vi "ex_GetOneLineFromChunk.vi"(8 "error in (no error)":errorcluster, 9 "file_params":T1 {"time preference" items=["Absolute", "Relative"]; "x_columns" items=["None", "One", "Multiple"]}, 10 "current chunk":string, 11 "file refs in":T2={"file ref"=refnum, "file size (bytes:0)"=0, "read pointer (bytes:0)"=0, "chunk size (bytes:65000)"=65000}) -> (0 "error out":errorcluster, 1 "line":string, 2 "chunk out":string, 3 "dup file refs":T2={"file ref"=refnum, "file size (bytes:0)"=0, "read pointer (bytes:0)"=0, "chunk size (bytes:65000)"=65000}, 4 "end-of-file?":bool)   [LabVIEW 2017]
uses:
  <vilib>/express/express shared/ExFile.llb/ex_FileReference.ctl
  <vilib>/express/express input/ExFileReadBlock.llb/ex_ReadFileParams.ctl
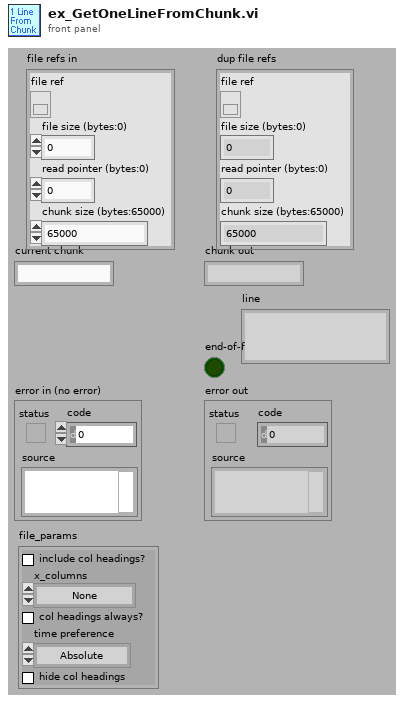
[diagram p1: front panel]
types:
  T1 = typedef "ex_ReadFileParams.ctl" = cluster{"include col headings?":bool, "x_columns":u16, "col headings always?":bool, "time preference":u16, "hide col headings":bool}
  T2 = typedef "ex_FileReference.ctl" = cluster{"file ref":refnum<file>, "file size (bytes:0)":i32, "read pointer (bytes:0)":i32, "chunk size (bytes:65000)":i32}
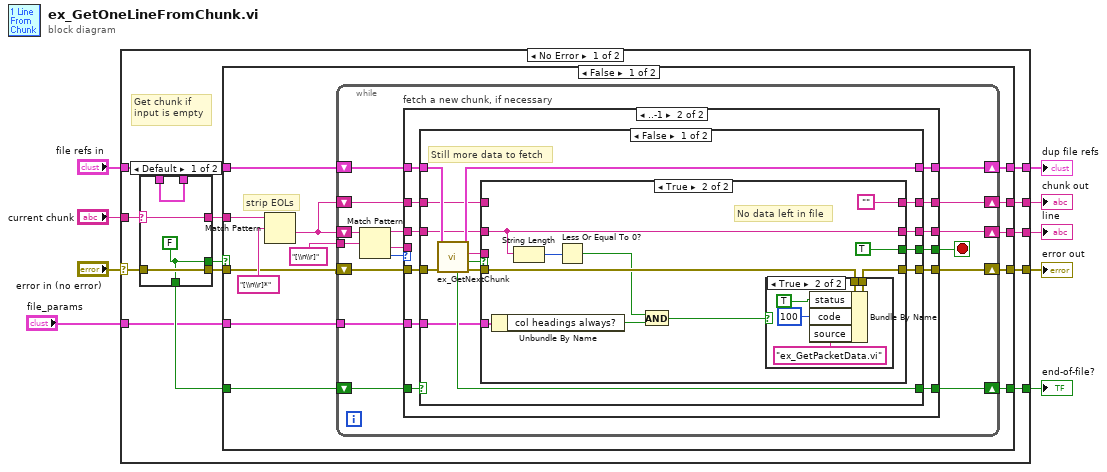
[diagram p0: block diagram]
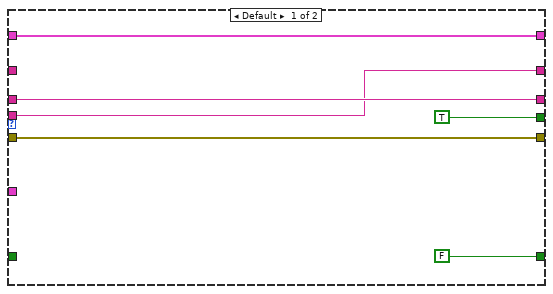
[diagram p2: hidden frame]
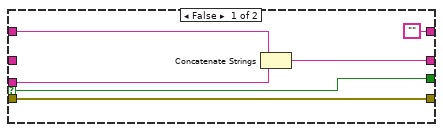
[diagram p3: hidden frame]
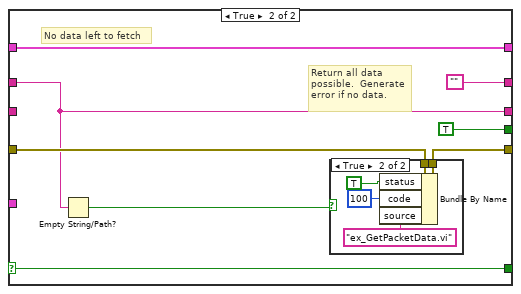
[diagram p5: hidden frame]
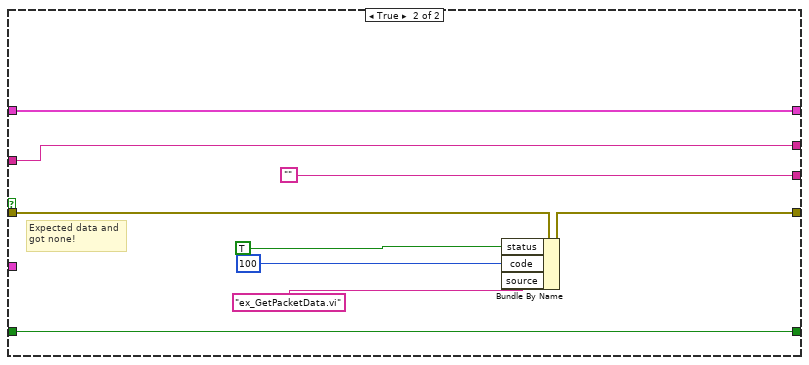
[diagram p7: hidden frame]
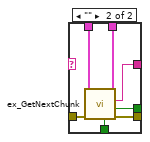
[diagram p8: hidden frame]
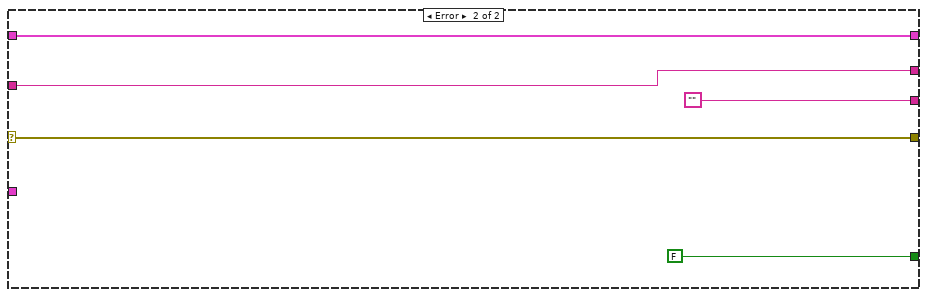
[diagram p9: hidden frame]
diagram:
  n1 = case shown="No Error" "error in (no error)" {
    selector: "error in (no error)" -> [w16 w144]
    tunnel: "current chunk" -> [w18 w145]
    tunnel: [w23 w145] -> w7
    tunnel: [w19 w144] -> w6
    tunnel: [w22 ""] -> w5
    tunnel: [w21 w143] -> w4
    tunnel: "file refs in" -> [w14 w143]
    tunnel: [w20 FALSE] -> w2
    tunnel: "file_params" -> [w10 _]
    frame No Error {
      # "Get chunk if\ninput is empty"
      n2 = case shown="Default" w18 {
        selector: w18 -> [w132 _]
        tunnel: [w132 w136] -> w17
        tunnel: w16 -> [w131 w140]
        tunnel: w14 -> [w133 w139]
        tunnel: [w133 w138] -> w15
        tunnel: [w131 w137] -> w13
        tunnel: [w130 w135] -> w12
        tunnel: [w130 w134] -> w11
        frame Default {
          w130 = FALSE ("no data error")
        }
        frame "" {
          n3 = call <vilib>:"ex_GetNextChunk.vi"("error in (no error)"=w140, "file refs"=w139) -> ("error out"=w137:errorcluster, "no data error"=w135:bool, "chunk"=w136:string, "dup file refs"=w138:T2, "end-of-file?"=w134:bool)  [unwired: 3 in, 2 out]
        }
      }
      n4 = case shown="False" w12 {
        tunnel: [w34 w122] -> w23
        tunnel: [w33 ""] -> w22
        tunnel: [w32 w123] -> w21
        tunnel: [w26 w124] -> w20
        tunnel: [w31 w125] -> w19
        tunnel: w17 -> [w29 w122]
        tunnel: w15 -> [w28 w123]
        tunnel: w13 -> [w27 w126]
        tunnel: w11 -> [w25 w124]
        tunnel: w10 -> [w24 _]
        frame False {
          # "strip EOLs"
          n5 = Match Pattern(string=w29, regular expression="[\\n\\r]*") -> (after substring=w36:string)  [unwired: 4 out]
          n6 = while {
            shift-right: [w44] -> w34
            shift-left: w36 -> [w47]
            shift-right: [w45] -> w33
            shift-left: w36 -> [w52]
            tunnel: "[\\n\\r]" -> [w51]
            shift-right: [w41] -> w31
            shift-left: w27 -> [w49]
            shift-right: [w48] -> w32
            shift-left: w28 -> [w42]
            shift-right: [w39] -> w26
            shift-left: w25 -> [w40]
            tunnel: w24 -> [w37]
            stop <- w38 stop-if-true
            n7 = Match Pattern(string=w52, regular expression=w51) -> (before substring=w46:string, after substring=w43:string, offset past match=w50:i32)  [unwired: 2 out]
            n8 = case "fetch a new chunk, if necessary" shown="..-1" w50 {
              tunnel: [w58 w66] -> w48
              tunnel: [w53 w70] -> w41
              tunnel: [TRUE w69] -> w38
              tunnel: w42 -> [w58 w67]
              tunnel: w49 -> [w53 w68]
              tunnel: w47 -> [_ w63]
              tunnel: w46 -> [w57 w64]
              tunnel: [w57 w61] -> w45
              tunnel: [w55 w62] -> w44
              tunnel: w43 -> [w55 _]
              tunnel: [FALSE ("end-of-file?") w65] -> w39
              tunnel: w40 -> [_ w60]
              tunnel: w37 -> [_ w59]
              frame Default {
              }
              frame ..-1 {
                n9 = case shown="False" w60 {
                  selector: w60 -> [_ w112]
                  tunnel: [w83 w113] -> w70
                  tunnel: [w82 TRUE] -> w69
                  tunnel: w68 -> [w81 w114]
                  tunnel: w67 -> [w78 w109]
                  tunnel: [w77 w109] -> w66
                  tunnel: [w76 w112] -> w65
                  tunnel: w64 -> [w75 _]
                  tunnel: w63 -> [w74 w107]
                  tunnel: [w73 ""] -> w62
                  tunnel: [w72 w107] -> w61
                  tunnel: w59 -> [w71 _]
                  frame False {
                    # "Still more data to fetch"
                    n10 = call <vilib>:"ex_GetNextChunk.vi"("error in (no error)"=w81, "file refs"=w78) -> ("error out"=w84:errorcluster, "no data error"=w79:bool, "chunk"=w80:string, "dup file refs"=w77:T2, "end-of-file?"=w76:bool)  [unwired: 3 in, 2 out]
                    n11 = case shown="True" w79 {
                      selector: w79 -> [w89 _]
                      tunnel: w84 -> [w90 w100]
                      tunnel: [w90 w99] -> w83
                      tunnel: [w89 TRUE] -> w82
                      tunnel: w80 -> [w88 _]
                      tunnel: w75 -> [_ w95]
                      tunnel: w74 -> [w86 _]
                      tunnel: ["" ""] -> w73
                      tunnel: [w85 w95] -> w72
                      tunnel: w71 -> [_ w96]
                      frame False {
                        n12 = Concatenate Strings(w86, w88) -> (w85:string)
                      }
                      frame True {
                        # "No data left in file"
                        n13 = Unbundle By Name(w96) -> ("col headings always?"=w93:bool)
                        n14 = String Length(string=w95) -> (length=w94:i32)
                        n15 = Less Or Equal To 0?(x=w94) -> (x <= 0?=w92:bool)
                        n16 = And(x=w92, y=w93) -> (x .and. y?=w91:bool)
                        n17 = case shown="True" w91 {
                          tunnel: w100 -> [w101 w106]
                          tunnel: [w101 w105] -> w99
                          frame False {
                          }
                          frame True {
                            n18 = Bundle By Name(cluster=w106, "status"=TRUE, "code"=100, "source"="ex_GetPacketData.vi") -> (w105:errorcluster)
                          }
                        }
                      }
                    }
                  }
                  frame True {
                    # "Return all data\npossible.  Generate\nerror if no data."
                    # "No data left to fetch"
                    n19 = Empty String/Path?(string/path=w107) -> (empty?=w108:bool)
                    n20 = case shown="True" w108 {
                      tunnel: w114 -> [w115 w120]
                      tunnel: [w115 w119] -> w113
                      frame False {
                      }
                      frame True {
                        n21 = Bundle By Name(cluster=w120, "status"=TRUE, "code"=100, "source"="ex_GetPacketData.vi") -> (w119:errorcluster)
                      }
                    }
                  }
                }
              }
            }
          }
        }
        frame True {
          # "Expected data and\ngot none!"
          n22 = Bundle By Name(cluster=w126, "status"=TRUE, "code"=100, "source"="ex_GetPacketData.vi") -> (w125:errorcluster)
        }
      }
    }
    frame Error {
    }
  }
  "chunk out" <- w7
  "end-of-file?" <- w2
  "error out" <- w6
  "line" <- w5
  "dup file refs" <- w4
